vi "TestKnifeEdgeMeasurement.vi"() -> ()   [LabVIEW 2018]
uses:
  Hardware Mfg/Thorlabs Translation Stages/Controls/Translation Stage Cluster.ctl
  General/Controls/Translation Stage Types.ctl
  General/Controls/Go Scan Actions.ctl
panel:
  out "size(s)":i32
  out "Waveform Chart":dbl(graph)
  in  "path":path=path "C:/Users/BOAS-USER/Documents/Data/0507/knifeedge"
  out "Current Position":cluster{"X":dbl, "Y":dbl}
  out "Power":dbl
  out "Current State":T1=enum."Init Scan Head"
  in  "X Stage":T2={"Position"=0.0, "Is.Enabled?"=TRUE, "Is.Connected?"=FALSE, "Device SN"="45876539", "AccelerationMaximum"=20.0, "VelocityMaximum"=20.0, "Acceleration"=10.0, "Velocity"=10.0, "waitTimeout (ms)"=10000, "Model"=enum."Thorlabs LTS", "Is.Homed?"=FALSE}
  in  "Y Stage":T2={"Position"=0.0, "Is.Enabled?"=TRUE, "Is.Connected?"=FALSE, "Device SN"="45876539", "AccelerationMaximum"=0.0, "VelocityMaximum"=0.0, "Acceleration"=0.0, "Velocity"=0.0, "waitTimeout (ms)"=10000, "Model"=enum."None", "Is.Homed?"=FALSE}
  in  "Mosaic Paramter":T4={"X Axis"={"Start [mm]"=20.0, "Steps [pts]"=100, "End [mm]"=25.0}, "Y Axis"={"Start [mm]"=0.0, "Steps [pts]"=1, "End [mm]"=0.0}, "Scan Pattern"=enum."Uni-directional", "Overlap Options"={"Overlap Type"=enum."No Overlap", "Percent Overlap"=0, "Justify"=enum."Start"}}
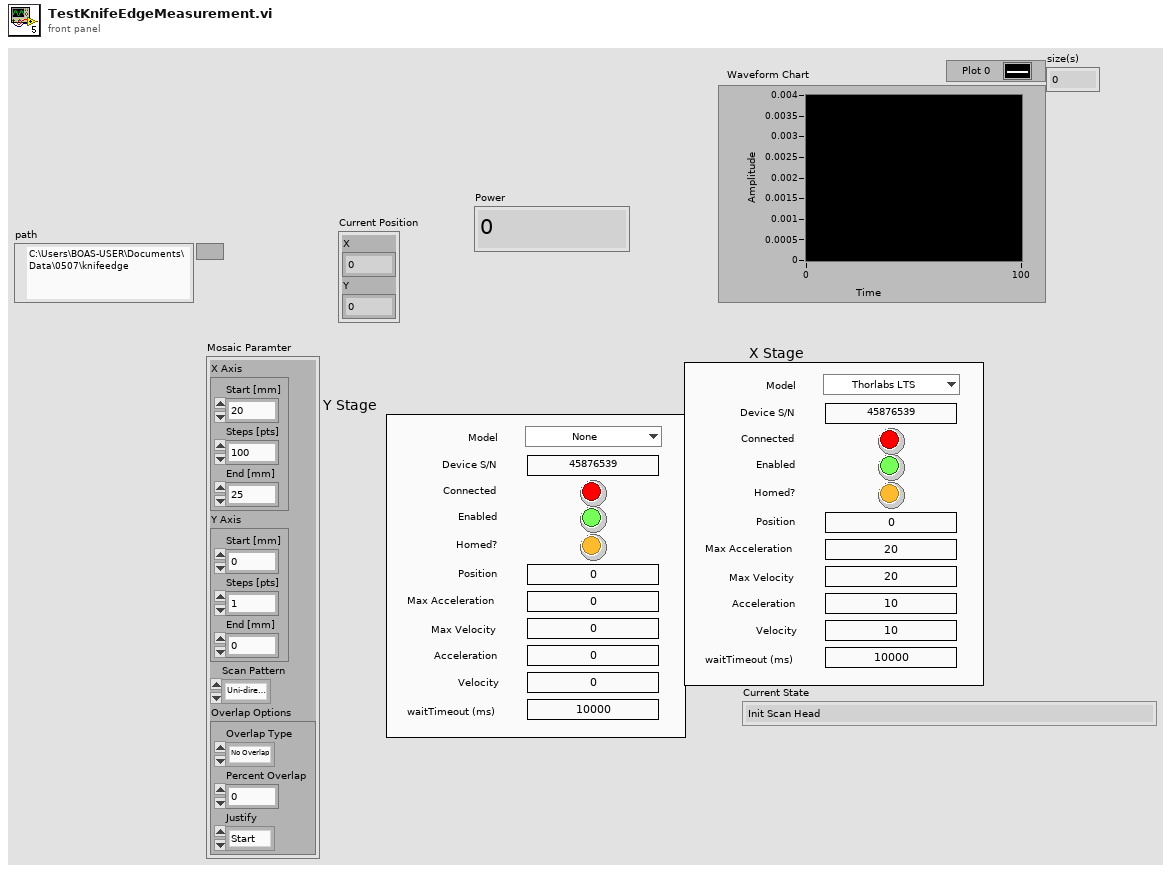
[diagram p1: front panel]
types:
  T1 = typedef "Go Scan Actions.ctl" = enum16{"Init", "Init Scan Head", "Init Table Stage", "Init Vibratome", "Generate Mosaic", "Go Image Home", "Go Mosaic", "Acquire Image", "Go Vibratome", "Slice", "Finished"}
  T2 = typedef "Translation Stage Cluster.ctl" = cluster{"Position":dbl, "Is.Enabled?":bool, "Is.Connected?":bool, "Device SN":string, "AccelerationMaximum":dbl, "VelocityMaximum":dbl, "Acceleration":dbl, "Velocity":dbl, "waitTimeout (ms)":i32, "Model":T3, "Is.Homed?":bool}
  T3 = typedef "Translation Stage Types.ctl" = enum16{"None", "Thorlabs LTS", "Thorlabs MLJ"}
  T4 = cluster{"X Axis":cluster{"Start [mm]":dbl, "Steps [pts]":u16, "End [mm]":dbl}, "Y Axis":cluster{"Start [mm]":dbl, "Steps [pts]":u16, "End [mm]":dbl}, "Scan Pattern":enum16{"Uni-directional", "Bi-Directional", "Spiral Out", "Spiral In"}, "Overlap Options":cluster{"Overlap Type":enum16{"No Overlap", "X Only", "Y Only", "X and Y"}, "Percent Overlap":u8, "Justify":enum16{"Start", "Center", "End"}}}
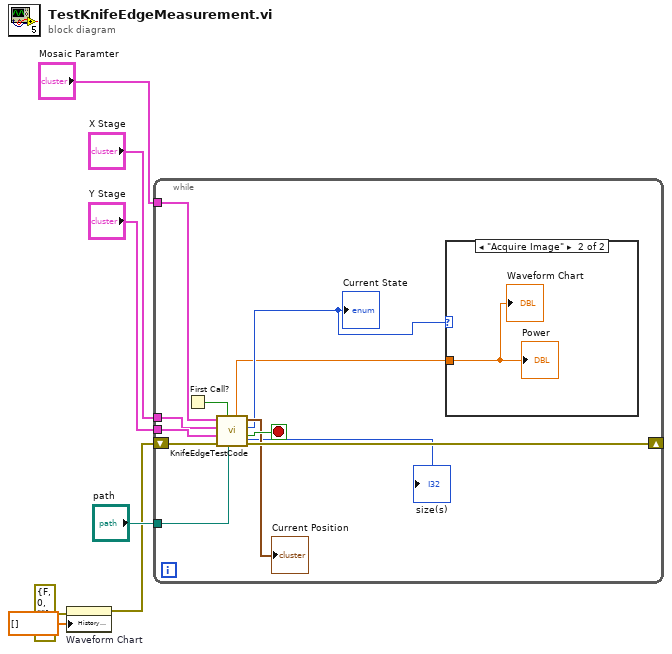
[diagram p0: block diagram]
diagram:
  n1 = property on="Waveform Chart" class="WFChart (strict)"(error in=errorcluster {"status"=FALSE, "code"=0, "source"=""} ("Error Out"), "History Data"=dbl[] []) -> (error out=w3:errorcluster)  [unwired: 1 in, 1 out]
  n2 = while {
    tunnel: "Mosaic Paramter" -> [w19]
    tunnel: "Y Stage" -> [w18]
    tunnel: "X Stage" -> [w17]
    shift-right: [w14] -> _
    shift-left: w3 -> [w13]
    tunnel: "path" -> [w11]
    stop <- w15 stop-if-true
    n3 = First Call?() -> (First Call?: T/F=w16:bool)
    n4 = call "KnifeEdgeTestCode.vi"("path"=w11, "Init"=w16, "Error In"=w13, "Z Stage"=w18, "X Stage"=w17, "Mosaic Paramter"=w19) -> ("Error Out"=w14:errorcluster, "Finished?"=w15:bool, "Current State"=w10:T1, "Current Position"=→"Current Position":cluster{"X":dbl, "Y":dbl}, "size(s)"=→"size(s)":i32, "Power"=w9:dbl)
    "Current State" <- w10
    n5 = case shown="\"Acquire Image\"" w10 {
      tunnel: w9 -> [_ w20]
      frame "Init", Default {
      }
      frame "Acquire Image" {
        "Power" <- w20
        "Waveform Chart" <- w20
      }
    }
  }
